vi "Timer_Initialize.vi"(8 "error in (no error)":errorcluster, 11 "Timer in":refnum<class "Timer.lvclass">) -> (0 "error out":errorcluster, 3 "Timer out":refnum<class "Timer.lvclass">)   [LabVIEW 2020, in "Timer.lvclass"]
doc: "Initialize Timer method"
uses:
  Timer.lvclass
  Timer.lvclass/Timer.ctl
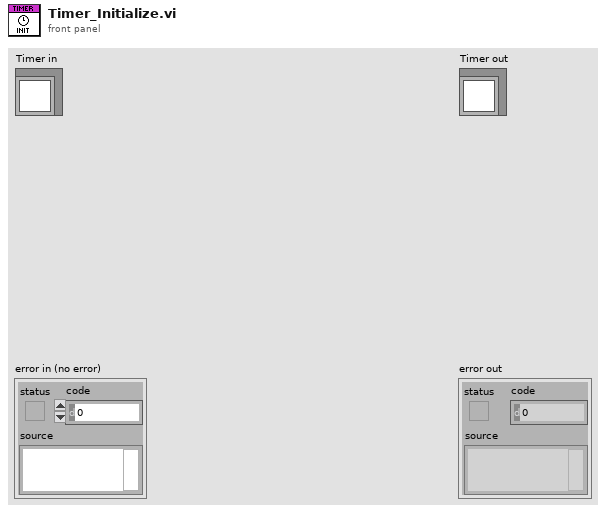
[diagram p1: front panel]
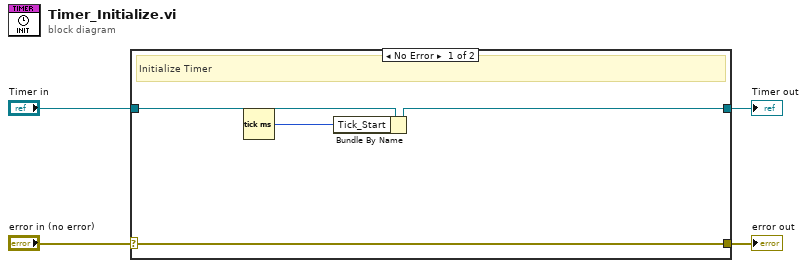
[diagram p0: block diagram]
diagram:
  n1 = case shown="No Error" "error in (no error)" {
    selector: "error in (no error)" -> [w7 w10]
    tunnel: [w7 w10] -> w3
    tunnel: [w6 w9] -> w1
    tunnel: "Timer in" -> [w8 w9]
    frame No Error {
      # "Initialize Timer"
      n2 = Tick Count (ms)() -> (millisecond timer value=w5:u32)
      n3 = Bundle By Name(cluster=w8, "Tick_Start"=w5) -> (w6:refnum<class "Timer.lvclass">)
    }
    frame Error {
    }
  }
  "error out" <- w3
  "Timer out" <- w1
